vi "Temp Moving Average.vi"(1 "PtByPt":dbl) -> (0 "Temperature":dbl)   [LabVIEW 2013, in "main.lvlib"]
uses:
  main.lvlib
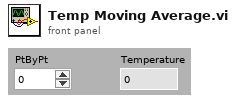
[diagram p1: front panel]
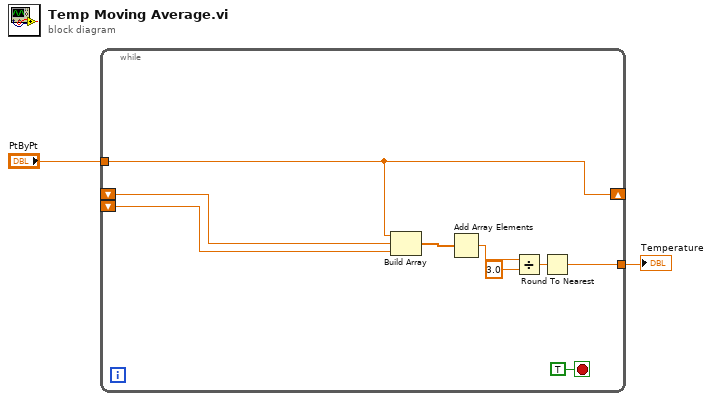
[diagram p0: block diagram]
diagram:
  n1 = while {
    shift-right: [w8] -> _
    shift-left: _ -> [w11]
    tunnel: [w10] -> w2
    tunnel: "PtByPt" -> [w8]
    shift-left: _ -> [w7]
    stop <- TRUE stop-if-true
    n2 = Build Array(w8, w11, w7) -> (w4:dbl[])
    n3 = Add Array Elements(numeric array=w4) -> (sum=w6:dbl)
    n4 = Divide(x=w6, y=3.0) -> (x/y=w5:dbl)
    n5 = Round To Nearest(number=w5) -> (nearest integer value=w10:dbl)
  }
  "Temperature" <- w2
